vi "test-DiffDriveSim-convergence.vi"() -> (3 "Test Passed":bool)   [LabVIEW 2019]
uses:
  <vilib>/Rock Robotics/WPI/ThirdParty/JAS_Junk/TrajLib/DCMOTOR.CTL
  <vilib>/Rock Robotics/WPI/ThirdParty/JAS_Junk/TrajLib/LINEAR_SYSTEM.ctl
  <vilib>/Analysis/Matrix/Datatypes/RealMatrix.ctl
  <vilib>/Rock Robotics/WPI/ThirdParty/JAS_Junk/TrajLib/DIFF_DRIVE_TRAIN_SIM.ctl
  <vilib>/Rock Robotics/WPI/ThirdParty/JAS_Junk/TrajLib/DIFF_DRIVE_ToughBoxMini_MotorChoice_ENUM.ctl
  <vilib>/Rock Robotics/WPI/ThirdParty/JAS_Junk/TrajLib/TRAJECTORY_SPLINE_TYPE_ENUM.ctl
  <vilib>/Rock Robotics/WPI/ThirdParty/JAS_Junk/TrajLib/Translation_Create.vi
  <vilib>/Rock Robotics/WPI/ThirdParty/JAS_Junk/TrajLib/Rotation_CreateAngle.vi
  <vilib>/Rock Robotics/WPI/ThirdParty/JAS_Junk/TrajLib/MatBuilder_Create.vi
  <vilib>/Rock Robotics/SystemInterfaces/NetworkCommunication/NetComm_UsageReport_report.vi
  <vilib>/Rock Robotics/WPI/ThirdParty/JAS_Junk/TrajLib/DiffDriveKinematicsConstraint_New.vi
  <vilib>/Rock Robotics/WPI/ThirdParty/JAS_Junk/TrajLib/MatBuilder_Fill.vi
  <vilib>/Rock Robotics/WPI/ThirdParty/JAS_Junk/TrajLib/MatrixHelper_Zero.vi
  <vilib>/Rock Robotics/WPI/ThirdParty/JAS_Junk/TrajLib/Util_CalcDist.vi
  <vilib>/Rock Robotics/WPI/ThirdParty/JAS_Junk/TrajLib/LinearSystem_New.vi
  <vilib>/Rock Robotics/WPI/ThirdParty/JAS_Junk/TrajLib/Util_LibraryGlobals.vi
  <vilib>/Rock Robotics/WPI/ThirdParty/JAS_Junk/TrajLib/Trajectory_Library.lvlib
  <vilib>/Analysis/Matrix/NI_Matrix.lvlib
panel:
  in  "Tab Control":T1(tab)
  out "Left Motor Vel (PV)":dbl format="%20.3f"
  out "Right Motor Vel (PV)":dbl format="%20.3f"
  out "CO Chart":cluster{"Voltage":dbl}(graph)
  out "PV Chart":T2(graph)
  out "Motor Amps":dbl format="%20.3f"
  out "Sim Upd Err":bool
  out "Lin Sys Size Cooerced":bool
  out "Pose Norm":dbl
  out "Pos Passed":bool
  out "DiffDriveMotor":T3 {"Jr_KgM2" format="%13.5p"; "L_H" format="%13.5p"; "Kt_NMPerAmp" format="%13.5p"; "KvINV_RadPerSecPerVolt" format="%13.5p"; "R_Ohms" format="%13.5p"; "FreeSpeed_RadPerSec" format="%13.5p"; "FreeCurrent_Amps" format="%13.5p"; "StallCurrent_Amps" format="%13.5p"; "StallTorque_NM" format="%13.5p"; "nominalVoltage_Volts" format="%13.5p"}
  out "m_DiffDriveVel":T4
  out "Differential Drive Train Sim":T6 {"m_Motor"."Jr_KgM2" format="%13.5p"; "m_Motor"."L_H" format="%13.5p"; "m_Motor"."Kt_NMPerAmp" format="%13.5p"; "m_Motor"."KvINV_RadPerSecPerVolt" format="%13.5p"; "m_Motor"."R_Ohms" format="%13.5p"; "m_Motor"."FreeSpeed_RadPerSec" format="%13.5p"; "m_Motor"."FreeCurrent_Amps" format="%13.5p"; "m_Motor"."StallCurrent_Amps" format="%13.5p"; "m_Motor"."StallTorque_NM" format="%13.5p"; "m_Motor"."nominalVoltage_Volts" format="%13.5p"}
  # "<States,States>"
  # "<States,Inputs>"
  # "<Outputs,States>"
  # "<Outputs,Inputs>"
  # "<States, 1>"
  # "<Outputs, 1>"
  # "<Inputs, 1>"
  # "<Outputs, 1>"
  # "<States,States>"
  # "<States,Inputs>"
  # "<Outputs,States>"
  # "<Outputs,Inputs>"
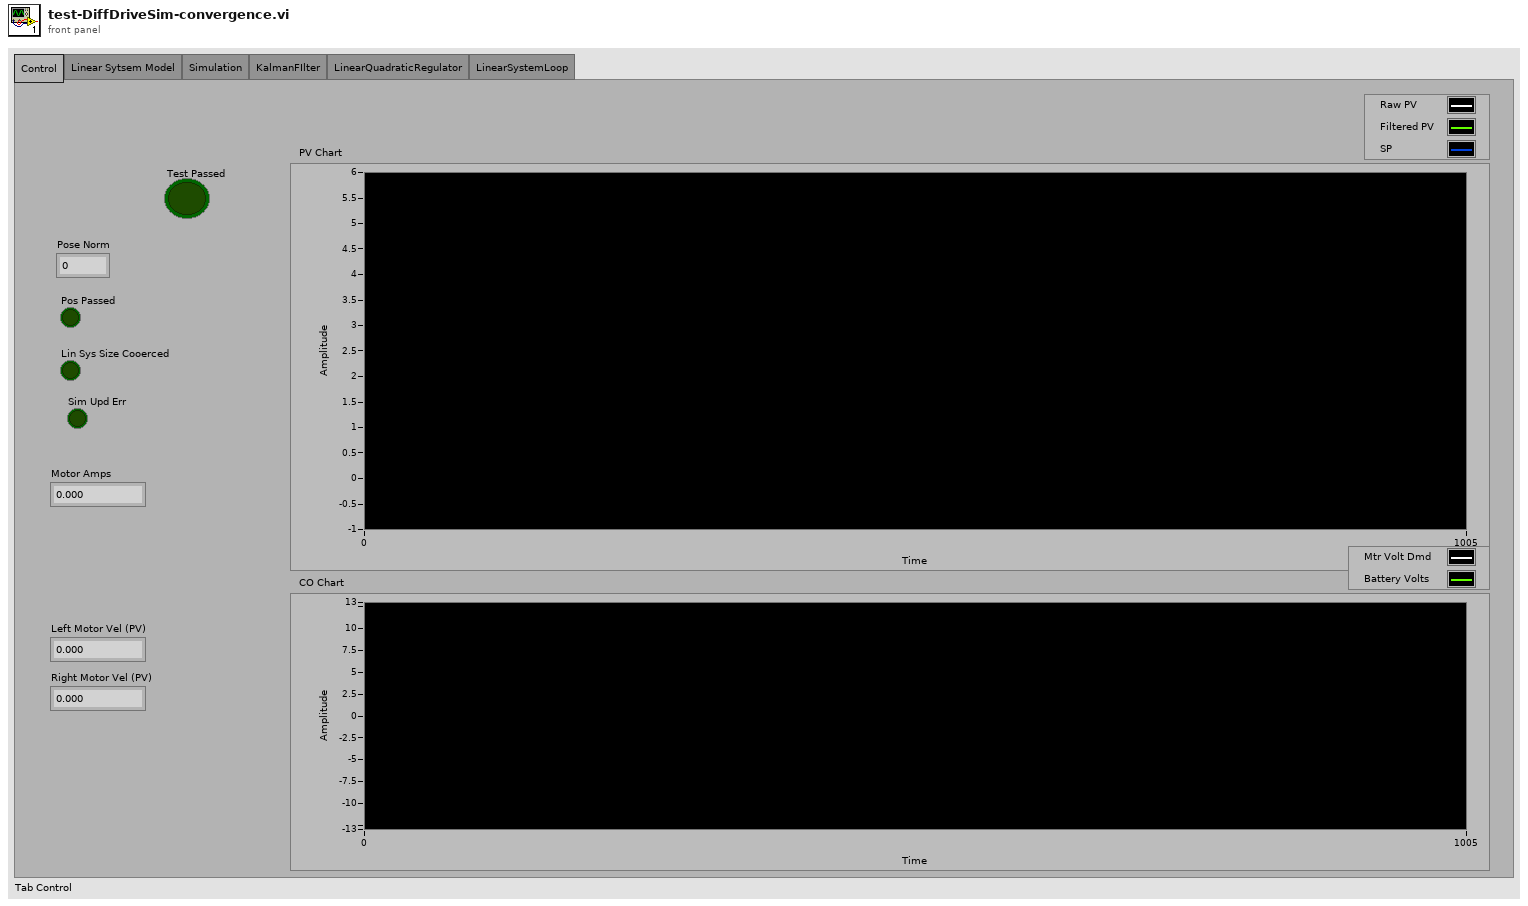
[diagram p1: front panel]
types:
  T1 = enum32{"Control", "Linear Sytsem Model", "Simulation", "KalmanFIlter", "LinearQuadraticRegulator", "LinearSystemLoop"}
  T2 = cluster{"LeftVelocity_M_Per_Sec":dbl, "RightVel_M_Per_Sec":dbl}
  T3 = typedef "Trajectory_Library.lvlib/DCMOTOR.CTL" = cluster{"nominalVoltage_Volts":dbl, "StallTorque_NM":dbl, "StallCurrent_Amps":dbl, "FreeCurrent_Amps":dbl, "FreeSpeed_RadPerSec":dbl, "R_Ohms":dbl, "KvINV_RadPerSecPerVolt":dbl, "Kt_NMPerAmp":dbl, "L_H":dbl, "Jr_KgM2":dbl}
  T4 = typedef "Trajectory_Library.lvlib/LINEAR_SYSTEM.ctl" = cluster{"m_A":T5, "m_B":T5, "m_C":T5, "m_D":T5, "States":i32, "Inputs":i32, "Outputs":i32}
  T5 = typedef "NI_Matrix.lvlib/RealMatrix.ctl" = dbl[][]
  T6 = typedef "Trajectory_Library.lvlib/DIFF_DRIVE_TRAIN_SIM.ctl" = cluster{"m_Plant":T4, "m_X":T5, "m_Y":T5, "m_U":T5, "MeasureStdDev":T5, "m_Motor":T3, "m_OriginalGearing":dbl, "m_CurrentGearing":dbl, "m_WheelRadius_M":dbl, "m_RB":dbl}
  T7 = typedef "Trajectory_Library.lvlib/TRAJECTORY_SPLINE_TYPE_ENUM.ctl" = enum16{"Cubic", "Cubic With Weights", "Quintic", "Quintic With Weights"}
  T8 = typedef "Trajectory_Library.lvlib/DIFF_DRIVE_ToughBoxMini_MotorChoice_ENUM.ctl" = enum16{"One CIM Per Side", "Two CIM Per Side", "One MiniCIM Per Side", "Two Mini CIM Per Side", "Two Falcon Per Side", "Two NEO Per Side"}
  T9 = typedef "Trajectory_Library.lvlib/TRAJ_CONFIG.ctl" = cluster{"MaxVelocity":dbl, "Max Acceleration":dbl, "StartVelocity":dbl, "End Velocity":dbl, "Reversed":bool, "DiffDrKineConstntDefined":bool, "CentAcellConstntDefined":bool, "DiffDrVoltConstntDefined":bool, "DIFF_DRIVE_KINE_CONSTRAINT":T10, "CENTRIPETAL_ACCEL_CONSTRAINT":T12, "SwerveDrKineConstntDefined":bool, "SWERVE_DRIVE_KINE_CONSTRAINT":T13, "DIFF_DRIVE_VOLTAGE_CONSTRAINT":T16, "MECANUM_DRIVE_KINE_CONSTRAINT":T18, "MecanumDrKineConstntDefined":bool}
  T10 = typedef "Trajectory_Library.lvlib/TRAJ_CONSTRAINT_DIIF_DRIVE_KINEMATICS.ctl" = cluster{"Max Speed (M/S)":dbl, "DIFF_DRIVE_KINEMATICS":T11, "Max Accel (M/S2)":dbl}
  T11 = typedef "Trajectory_Library.lvlib/DIFF_DRIVE_KINEMATICS.ctl" = cluster{"TrackWidth_Meters":dbl}
  T12 = typedef "Trajectory_Library.lvlib/TRAJ_CONSTRAINT_CENTRIPETAL_ACCEL.ctl" = cluster{"Max Cent Accel":dbl}
  T13 = typedef "Trajectory_Library.lvlib/TRAJ_CONSTRAINT_SWERVE_DRIVE_KINEMATICS.ctl" = cluster{"Max Speed (M/S)":dbl, "SwerveKinematics":T14}
  T14 = typedef "Trajectory_Library.lvlib/SWERVE_DRIVE_KINEMATICS.ctl" = cluster{"NumModules":i32, "InverseKinematics":T5, "ForwardKinematics":T5, "Modules":T15[], "PrevCoR":T15}
  T15 = typedef "Trajectory_Library.lvlib/TRANSLATION2D.ctl" = cluster{"X":dbl, "Y":dbl}
  T16 = typedef "Trajectory_Library.lvlib/TRAJ_CONSTRAINT_DIIF_DRIVE_VOLTAGE.ctl" = cluster{"Max Voltage":dbl, "DIFF_DRIVE_KINEMATICS":T11, "SIMPLE_MOTOR_FF":T17}
  T17 = typedef "Trajectory_Library.lvlib/SIMPLE_MOTOR_FF.ctl" = cluster{"Ks":dbl, "Kv":dbl, "Ka":dbl}
  T18 = typedef "Trajectory_Library.lvlib/TRAJ_CONSTRAINT_MECA_DRIVE_KINEMATICS.ctl" = cluster{"Max Speed (M/S)":dbl, "MECA_DRIVE_KINEMATICS":T19}
  T19 = typedef "Trajectory_Library.lvlib/MECA_DRIVE_KINEMATICS.ctl" = cluster{"FrontLeft":T15, "FrontRight":T15, "RearLeft":T15, "RearRight":T15, "InverseKinematics":T5, "ForwardKinematics":T5, "PrevCoR":T15}
  T20 = typedef "Trajectory_Library.lvlib/WEIGHTED_WAYPOINT.ctl" = cluster{"TRANSLATION":T15, "ROTATION":T21, "SCALAR":dbl}
  T21 = typedef "Trajectory_Library.lvlib/ROTATION2D.ctl" = cluster{"VALUE":dbl, "COS":dbl, "SIN":dbl}
  T22 = typedef "Trajectory_Library.lvlib/TRAJECTORY.ctl" = cluster{"TotalTImeSecs":dbl, "States":T23[]}
  T23 = typedef "Trajectory_Library.lvlib/TRAJ_STATE.ctl" = cluster{"TimeSeconds":dbl, "Velocity":dbl, "Acceleration":dbl, "POSE":T24, "Curvature":dbl}
  T24 = typedef "Trajectory_Library.lvlib/POSE2D.ctl" = cluster{"TRANSLATION":T15, "ROTATION":T21}
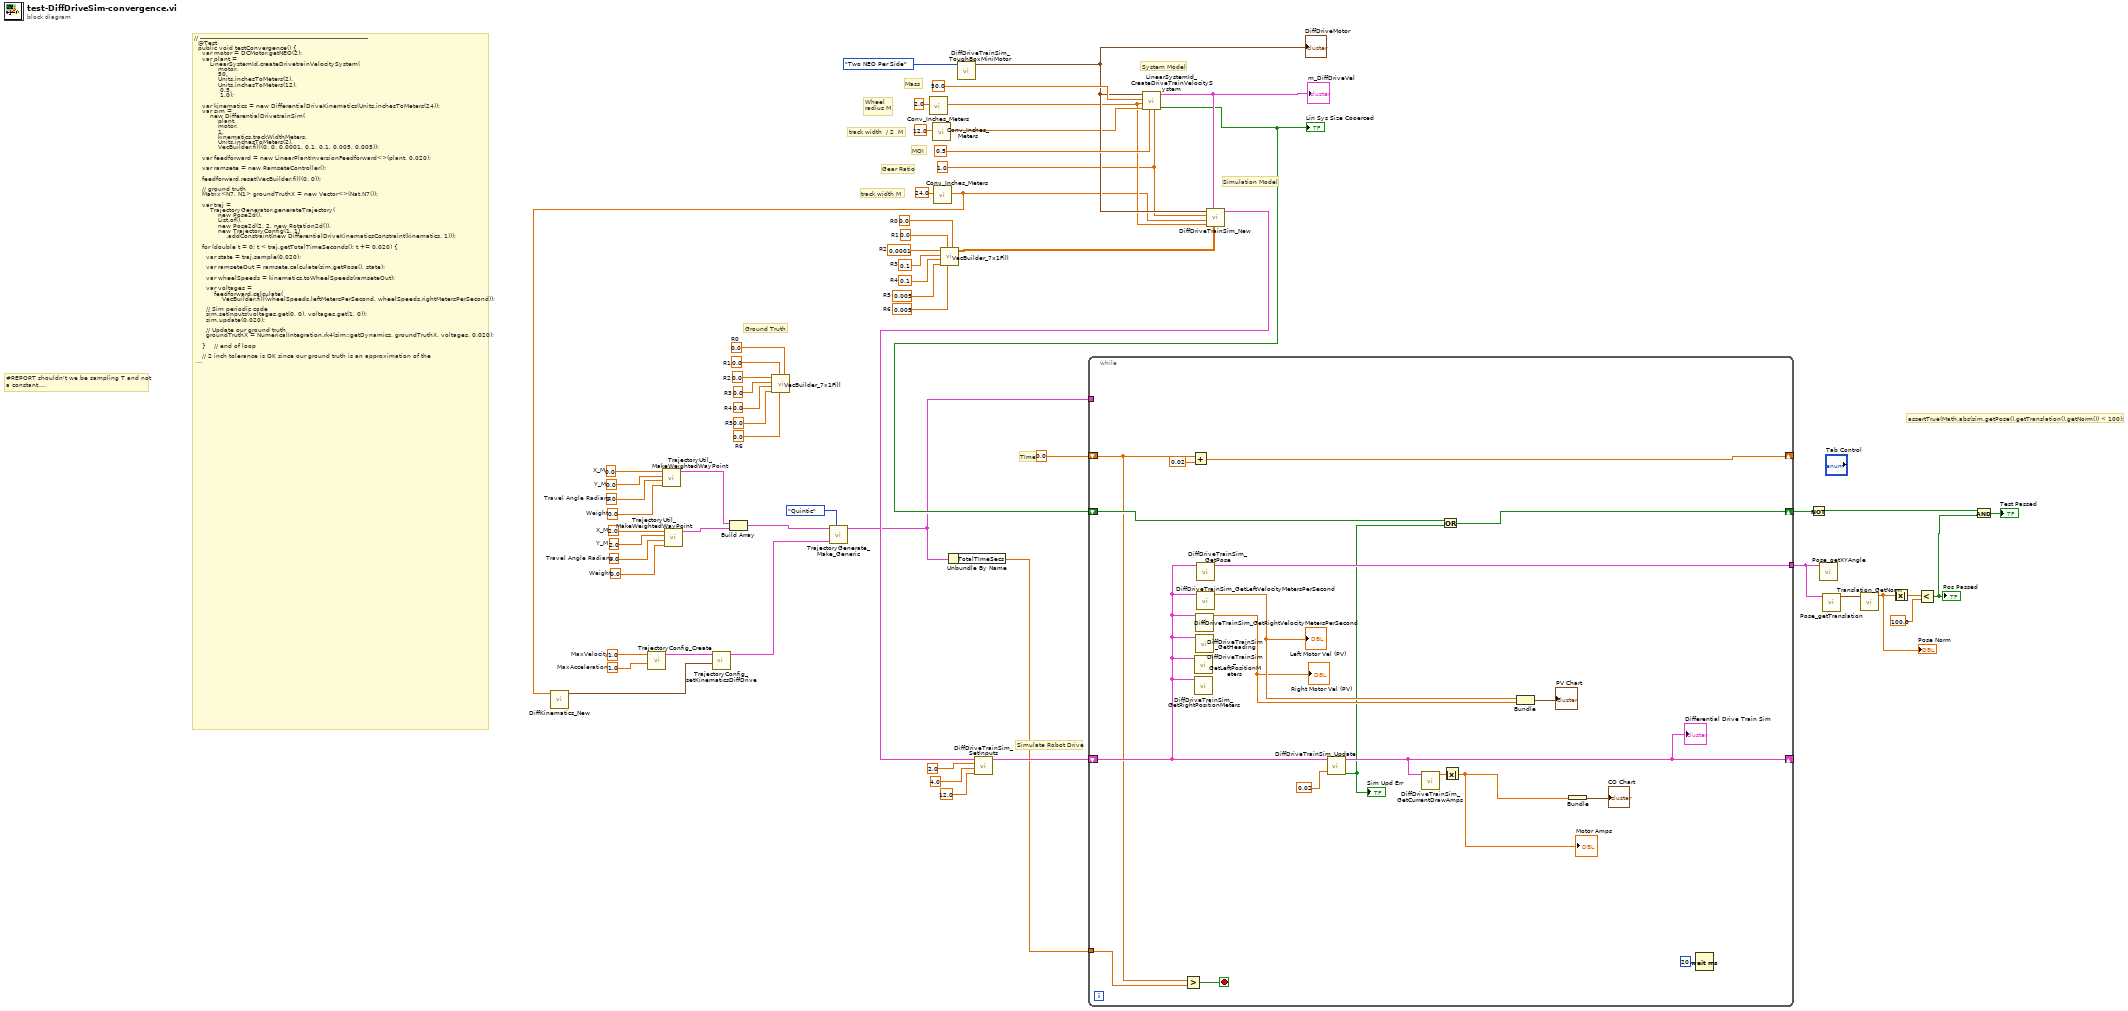
[diagram p0: block diagram]
diagram:
  w20 = 2.0  # X_M
  w19 = 2.0  # Y_M
  w18 = 0.0  # Travel Angle Radians
  w17 = 0.0  # Weight
  w16 = 0.0  # X_M
  w15 = 0.0  # Y_M
  w14 = 0.0  # Travel Angle Radians
  w13 = 0.0  # Weight
  w12 = 1.0  # MaxVelocity
  w11 = 1.0  # MaxAcceleration
  w28 = 0.0  # R6
  w27 = 0.0  # R5
  w26 = 0.0  # R4
  w25 = 0.0  # R3
  w24 = 0.0  # R2
  w23 = 0.0  # R1
  w22 = 0.0  # R0
  w51 = 0.005  # R6
  w50 = 0.005  # R5
  w49 = 0.1  # R4
  w48 = 0.1  # R3
  w47 = 0.0001  # R2
  w46 = 0.0  # R1
  w45 = 0.0  # R0
  w53 = 1.0 ("G")
  # "#REPORT shouldn't we be sampling T and not\na constant...."
  # "TIme"
  # "Ground Truth"
  # "// ------------------------------------------------------------------------------------\n  @Test\n  public void testConvergence() {\n    var motor = DCMotor.getNEO(2);\n    var plant =\n        LinearSystemId.createDrivetrainVelocitySystem(\n            motor, \n            50, \n            Units.inchesToMeters(2), \n            Units.inchesToMeters(12), \n             0.5, \n             1.0);\n\n    var kinematics = new DifferentialDriveKinematics(Units.inchesToMeters(24));\n    var sim =\n        new DifferentialDrivetrainSim(\n            plant,\n            motor,\n            1,\n            kinematics.trackWidthMeters,\n            Units.inchesToMeters(2),\n            VecBuilder.fill(0, 0, 0.0001, 0.1, 0.1, 0.005, 0.005));\n\n    var feedforward = new LinearPlantInversionFeedforward<>(plant, 0.020);\n\n    var ramsete = new RamseteController();\n\n    feedforward.reset(VecBuilder.fill(0, 0));\n\n    // ground truth\n    Matrix<N7, N1> groundTruthX = new Vector<>(Nat.N7());\n\n    var traj =\n        TrajectoryGenerator.generateTrajectory(\n            new Pose2d(),\n            List.of(),\n            new Pose2d(2, 2, new Rotation2d()),\n            new TrajectoryConfig(1, 1)\n                .addConstraint(new DifferentialDriveKinematicsConstraint(kinematics, 1)));\n\n    for (double t = 0; t < traj.getTotalTimeSeconds(); t += 0.020) {\n\n      var state = traj.sample(0.020);\n\n      var ramseteOut = ramsete.calculate(sim.getPose(), state);\n\n      var wheelSpeeds = kinematics.toWheelSpeeds(ramseteOut);\n\n      var voltages =\n          feedforward.calculate(\n              VecBuilder.fill(wheelSpeeds.leftMetersPerSecond, wheelSpeeds.rightMetersPerSecond));\n\n      // Sim periodic code\n      sim.setInputs(voltages.get(0, 0), voltages.get(1, 0));\n      sim.update(0.020);\n\n      // Update our ground truth\n      groundTruthX = NumericalIntegration.rk4(sim::getDynamics, groundTruthX, voltages, 0.020);\n\n    }    // end of loop\n\n    // 2 inch tolerance is OK since our ground truth is an approximation of the\n    // ODE solution using RK4 anyway\n    assertEquals(\n        groundTruthX.get(DifferentialDrivetrainSim.State.kX.value, 0),\n        sim.getState(DifferentialDrivetrainSim.State.kX),\n        0.05);\n    assertEquals(\n        groundTruthX.get(DifferentialDrivetrainSim.State.kY.value, 0),\n        sim.getState(DifferentialDrivetrainSim.State.kY),\n        0.05);\n    assertEquals(\n        groundTruthX.get(DifferentialDrivetrainSim.State.kHeading.value, 0),\n        sim.getState(DifferentialDrivetrainSim.State.kHeading),\n        0.01);\n  }\n\n\n}"
  # "assertTrue(Math.abs(sim.getPose().getTranslation().getNorm()) < 100);"
  # "track width M"
  # "Gear Ratio"
  # "Wheel\nradius M"
  # "track width  / 2  M"
  # "MOI"
  # "Simulation Model"
  # "System Model"
  # "Mass"
  # "Simulate Robot Drive"
  n1 = call <vilib>:"TrajectoryConfig_Create.vi"("MaxAcceleration"=w11, "MaxVelocity"=w12) -> ("TRAJECTORY_CONFIG"=w5:T9)  [unwired: 9 in]
  n2 = call <vilib>:"TrajectoryUtil_MakeWeightedWayPoint.vi"("Weight"=w13, "Travel Angle Radians"=w14, "Y_M"=w15, "X_M"=w16) -> ("WEIGHTED_WAYPOINT"=w8:T20)  [unwired: 7 in]
  n3 = call <vilib>:"TrajectoryUtil_MakeWeightedWayPoint.vi"("Weight"=w17, "Travel Angle Radians"=w18, "Y_M"=w19, "X_M"=w20) -> ("WEIGHTED_WAYPOINT"=w21:T20)  [unwired: 7 in]
  n4 = Build Array(w8, w21) -> (w9:T20[])
  n5 = call <vilib>:"VecBuilder_7x1Fill.vi"("R0"=w22, "R6"=w28, "R1"=w23, "R5"=w27, "R4"=w26, "R3"=w25, "R2"=w24) -> ()  [unwired: 4 in, 1 out]
  n6 = call <vilib>:"Conv_Inches_Meters.vi"("INCH"=2.0) -> ("Meters"=w55:dbl)  [unwired: 10 in]
  n7 = call <vilib>:"Conv_Inches_Meters.vi"("INCH"=12.0) -> ("Meters"=w56:dbl)  [unwired: 10 in]
  n8 = call <vilib>:"Conv_Inches_Meters.vi"("INCH"=24.0) -> ("Meters"=w7:dbl)  [unwired: 10 in]
  n9 = call <vilib>:"DiffKinematics_New.vi"("TrackWidth_Meters"=w7) -> ("DIFF_DRIVE_KINEMATICS"=w6:T11)  [unwired: 10 in]
  n10 = call <vilib>:"TrajectoryConfig_setKinematicsDiffDrive.vi"("DIFF_DRIVE_KINEMATICS"=w6, "inTRAJECTORY_CONFIG"=w5) -> ("outTRAJECTORY_CONFIG"=w4:T9)  [unwired: 9 in]
  n11 = call <vilib>:"TrajectoryGenerate_Make_Generic.vi"("Spline Type"=TRAJECTORY_SPLINE_TYPE_ENUM."Quintic", "traj_config"=w4, "WeightedWayPoints"=w9) -> ("TRAJECTORY"=w2:T22)  [unwired: 7 in, 1 out]
  n12 = call <vilib>:"VecBuilder_7x1Fill.vi"("R0"=w45, "R6"=w51, "R1"=w46, "R5"=w50, "R4"=w49, "R3"=w48, "R2"=w47) -> ("output matrix"=w44:T5)  [unwired: 4 in]
  n13 = Unbundle By Name(w2) -> ("TotalTImeSecs"=w1:dbl)
  n14 = call <vilib>:"DiffDriveTrainSim_ToughBoxMiniMotor.vi"("ToughBoxMiniMotor"=DIFF_DRIVE_ToughBoxMini_MotorChoice_ENUM."Two NEO Per Side") -> ("DriveMotor"=w57:T3)  [unwired: 10 in]
  "DiffDriveMotor" <- w57
  n15 = call <vilib>:"LinearSystemId_CreateDriveTrainVelocitySystem.vi"("G"=w53, "JKgMetersSquared"=0.5 ("Mass_Kg"), "rbMeters"=w56, "rMeters"=w55, "MassKg"=50.0 ("Mass_Kg"), "Motor"=w57) -> ("Size Coerced"=w33:bool, "Linearsystem"=w54:T4)  [unwired: 4 in]
  "m_DiffDriveVel" <- w54
  "Lin Sys Size Cooerced" <- w33
  n16 = call <vilib>:"DiffDriveTrainSim_New.vi"("MeasurementStdDev"=w44, "DriveTrainPlant"=w54, "WheelRadius_M"=w55, "TrackWidth_M"=w7, "Gearing"=w53, "DriveMotor"=w57) -> ("DiffDriveTrainSim"=w43:T6)  [unwired: 5 in]
  n17 = call <vilib>:"DiffDriveTrainSim_SetInputs.vi"("BatteryVoltage"=12.0, "Right_Volts"=4.0, "Left_Volts"=2.0, "in DiffDriveTrainSim"=w43) -> ("out DiffDriveTrainSim"=w42:T6)  [unwired: 6 in, 1 out]
  n18 = while {
    shift-right: [w78] -> _
    shift-left: w42 -> [w76]
    tunnel: [w70] -> w38
    shift-right: [w67] -> w32
    shift-left: w33 -> [w68]
    tunnel: w2 -> [_]
    shift-right: [w63] -> _
    shift-left: 0.0 -> [w65]
    tunnel: w1 -> [w66]
    stop <- w74 stop-if-true
    n19 = Greater?(x=w65, y=w66) -> (0:w74:bool)
    n20 = Add(x=w65, y=0.02) -> (x+y=w63:dbl)
    n21 = call <vilib>:"DiffDriveTrainSim_GetLeftPositionMeters.vi"("DiffDriveTrainSim"=w76) -> ()  [unwired: 10 in, 1 out]
    n22 = call <vilib>:"DiffDriveTrainSim_GetRightPositionMeters.vi"("DiffDriveTrainSim"=w76) -> ()  [unwired: 10 in, 1 out]
    n23 = call <vilib>:"DiffDriveTrainSim_GetHeading.vi"("DiffDriveTrainSim"=w76) -> ()  [unwired: 10 in, 1 out]
    n24 = call <vilib>:"DiffDriveTrainSim_GetRightVelocityMetersPerSecond.vi"("DiffDriveTrainSim"=w76) -> ("RightVel_M_Per_Sec"=w72:dbl)  [unwired: 10 in]
    "Right Motor Vel (PV)" <- w72
    n25 = call <vilib>:"DiffDriveTrainSim_GetPose.vi"("DiffDriveTrainSim"=w76) -> ("Pose"=w70:T24)  [unwired: 10 in]
    n26 = call <vilib>:"DiffDriveTrainSim_GetLeftVelocityMetersPerSecond.vi"("DiffDriveTrainSim"=w76) -> ("LeftVelocity_M_Per_Sec"=w77:dbl)  [unwired: 10 in]
    "Left Motor Vel (PV)" <- w77
    n27 = call <vilib>:"DiffDriveTrainSim_Update.vi"("dT_Seconds"=0.02, "in DiffDriveTrainSim"=w76) -> ("Error"=w69:bool, "out DiffDriveTrainSim"=w78:T6)  [unwired: 8 in]
    "Sim Upd Err" <- w69
    "Differential Drive Train Sim" <- w78
    n28 = call <vilib>:"DiffDriveTrainSim_GetCurrentDrawAmps.vi"("DiffDriveTrainSim"=w78) -> ("TotalCurrent_Amps"=w79:dbl)  [unwired: 10 in]
    n29 = Or(x=w68, y=w69) -> (x .or. y?=w67:bool)
    n30 = Absolute Value(x=w79) -> (abs(x)=w73:dbl)
    "Motor Amps" <- w73
    n31 = Bundle("LeftVelocity_M_Per_Sec"=w77, "RightVel_M_Per_Sec"=w72) -> (→"PV Chart":T2)  [unwired: 1 in]
    n32 = Bundle(w73) -> (→"CO Chart":cluster{dbl})  [unwired: 1 in]
    n33 = Wait (ms)(milliseconds to wait=u32 20) -> ()  [unwired: 1 out]
  }
  n34 = Not(x=w32) -> (.not. x?=w31:bool)
  n35 = call <vilib>:"Pose_getXYAngle.vi"("in POSE"=w38) -> ()  [unwired: 8 in, 3 out]
  n36 = call <vilib>:"Pose_getTranslation.vi"("in POSE"=w38) -> ("outTRANSLATION"=w37:T15)  [unwired: 10 in]
  n37 = call <vilib>:"Translation_GetNorm.vi"("In Translation"=w37) -> ("Norm"=w36:dbl)  [unwired: 10 in]
  "Pose Norm" <- w36
  n38 = Absolute Value(x=w36) -> (abs(x)=w35:dbl)
  n39 = Less?(x=w35, y=100.0) -> (x < y?=w30:bool)
  "Pos Passed" <- w30
  n40 = And(x=w31, y=w30) -> (x .and. y?=→"Test Passed":bool)
